vi "Check Element Description.vi"(7 "VolatusAPI":refnum<class "VolatusAPI.lvclass">, 8 "error in (no error)":errorcluster, 10 "Ref":refnum<vi>) -> (0 "error out":errorcluster, 1 "Register":bool, 3 "Element":refnum<class "GUI Element.lvclass">)   [LabVIEW 2020, in "VolatusGUI.lvlib" / "PluginGUI.lvclass"]
uses:
  PluginGUI.lvclass
  GUI Element/GUI Element.lvclass
  Volatus/VolatusAPI/VolatusAPI.lvclass
  PluginGUI.lvclass/PluginGUI.ctl
  VolatusGUI.lvlib
  volatus-gui-controls/VolatusGUIControls/VolatusGUIControls.lvlib
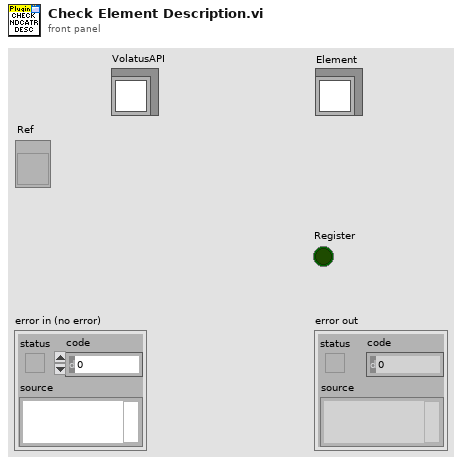
[diagram p1: front panel]
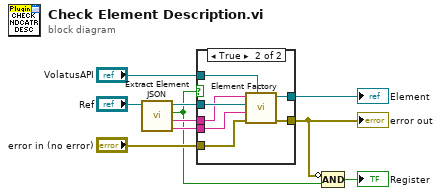
[diagram p0: block diagram]
diagram:
  n1 = call "Extract Element JSON.vi"("Ctl Refnum in"="Ref") -> ("JSON"=w2:string, "Type"=w3:string, "Is GUI Element"=w1:bool, "Ctl Refnum"=w4:refnum<vi>)  [unwired: 7 in]
  n2 = case shown="True" w1 {
    tunnel: [_ w18] -> w9
    tunnel: [w11 w17] -> w7
    tunnel: "VolatusAPI" -> [_ w16]
    tunnel: w4 -> [_ w15]
    tunnel: w3 -> [_ w14]
    tunnel: w2 -> [_ w13]
    tunnel: "error in (no error)" -> [w11 w12]
    frame False {
    }
    frame True {
      n3 = call "Element Factory.vi"("VolatusAPI"=w16, "error in (no error)"=w12, "JSON"=w13, "Ref"=w15, "Element Type"=w14) -> ("error out"=w17:errorcluster, "GUI Element"=w18:refnum<class "GUI Element.lvclass">)  [unwired: 5 in]
    }
  }
  "error out" <- w7
  "Element" <- w9
  n4 = Compound Arithmetic op=AND(invert w7, w1) -> (→"Register":bool)
